vi "Acknowledge Itetations End.vi"(8 "error in (no error)":errorcluster, 11 "Abstract Iterator Actor in":refnum<class "Abstract Iterator Actor.lvclass">) -> (0 "error out":errorcluster, 3 "Abstract Iterator Actor out":refnum<class "Abstract Iterator Actor.lvclass">)   [LabVIEW 2023, in "Iterator Actor.lvlib" / "Abstract Iterator Actor.lvclass"]
uses:
  Abstract Iterator Actor.lvclass
  Abstract Iterator Actor.lvclass/Abstract Iterator Actor.ctl
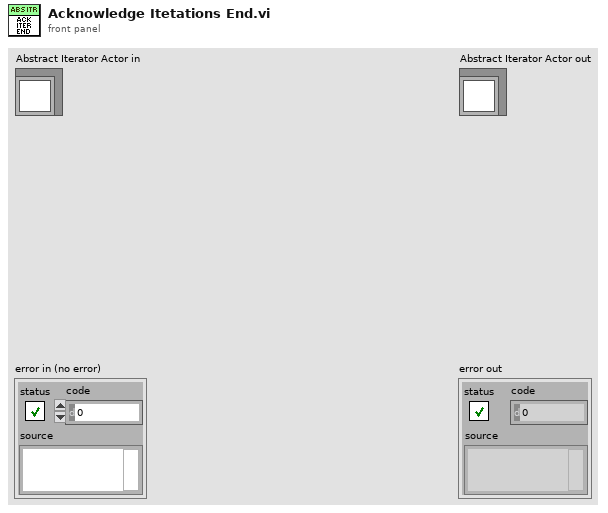
[diagram p1: front panel]
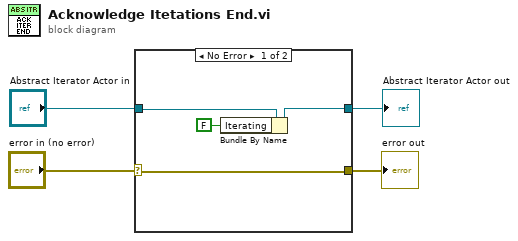
[diagram p0: block diagram]
diagram:
  n1 = case shown="No Error" "error in (no error)" {
    selector: "error in (no error)" -> [w7 w10]
    tunnel: [w7 w10] -> w3
    tunnel: [w6 w9] -> w1
    tunnel: "Abstract Iterator Actor in" -> [w8 w9]
    frame No Error {
      n2 = Bundle By Name(cluster=w8, "Iterating"=FALSE) -> (w6:refnum<class "Abstract Iterator Actor.lvclass">)
    }
    frame Error {
    }
  }
  "error out" <- w3
  "Abstract Iterator Actor out" <- w1
